vi "Median Filtering.vi"() -> ()   [LabVIEW 2020]
doc: "Uses the Median Filter VI to analyze pulses in the presence of noise. The example generates a pulse contaminated with Gaussian noise and applies a median filter. For comparison purposes, the VI computes the pulse parameters of the filtered pulse."
uses:
  <vilib>/Analysis/NI_AALPro.lvlib
  <vilib>/Analysis/NI_AALBase.lvlib
panel:
  in  "seed":i32=-1
  in  "Stop":bool
  out "Amplitude (est)":dbl format="%#.2g"
  in  "Amplitude":dbl=5.0 format="%#.6g"
  out "Delay (est)":dbl format="%#.2g"
  in  "Delay (samples)":i32=64
  out "Width (est)":dbl format="%#.2g"
  in  "Width (samples)":i32=32
  out "Waveform Graph":dbl[][](graph)
  in  "Gaussian noise sigma":dbl(slide)=0.8 scale=0.0..2.0
  in  "Filter rank":i32(slide)=7 scale=0.0..30.0
  in  "Samples":i32=128
  # "Overview: Demonstrates the application of a median filter on a noisy pulse.\nRequirements: LabVIEW Full Development System\nInstructions: \n1. Run the VI.\n2. Change the Gaussian noise sigma and Filter rank sliders and observe the effect on the estimated Amplitude, Width, and Delay.\n3. Change the seed value to generate different noise values.\n4. Click Stop to stop the VI."
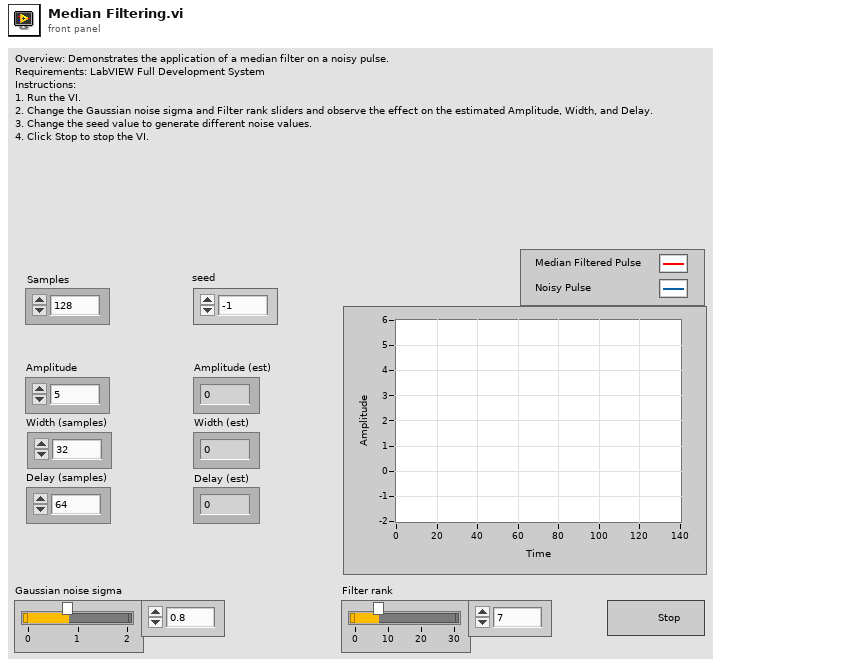
[diagram p1: front panel]
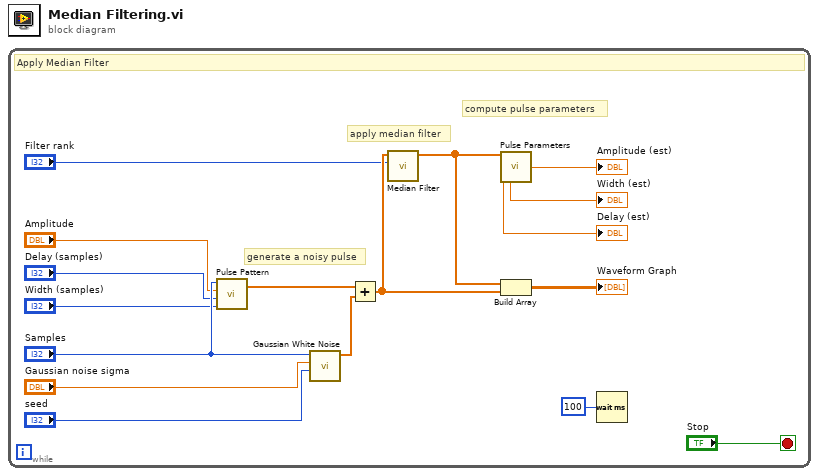
[diagram p0: block diagram]
diagram:
  n1 = while {
    stop <- "Stop" stop-if-true
    # "generate a noisy pulse"
    # "apply median filter"
    # "compute pulse parameters"
    # "Apply Median Filter"
    n2 = call <vilib>:"Pulse Pattern.vi"("width"="Width (samples)", "delay"="Delay (samples)", "amplitude"="Amplitude", "samples"="Samples") -> ("Pulse Pattern"=w9:dbl[])  [unwired: 1 out]
    n3 = call <vilib>:"Gaussian White Noise.vi"("seed"="seed", "standard deviation"="Gaussian noise sigma", "samples"="Samples") -> ("Gaussian noise pattern"=w16:dbl[])  [unwired: 7 in, 1 out]
    n4 = Add(x=w9, y=w16) -> (x+y=w7:dbl[])
    n5 = call <vilib>:"Median Filter.vi"("left rank"="Filter rank", "X"=w7) -> ("Filtered X"=w1:dbl[])  [unwired: 8 in, 1 out]
    n6 = call <vilib>:"Pulse Parameters.vi"("X"=w1) -> ("amplitude"=→"Amplitude (est)":dbl, "delay"=→"Delay (est)":dbl, "duration"=→"Width (est)":dbl)  [unwired: 4 in, 8 out]
    n7 = Build Array(w1, w7) -> (→"Waveform Graph":dbl[][])
    n8 = Wait (ms)(milliseconds to wait=u32 100) -> ()  [unwired: 1 out]
  }
